vi "Get Available Sets Extended.vi"(8 "error in (no error)":errorcluster, 10 "Item Types (all visible)":T1 items=["all visible", "all including hidden", "standard only", "startup only"], 11 "Session in":refnum<k21>) -> (0 "error out":errorcluster, 2 "Software Sets":T2[](array[typedef]) {"Items"."Visibility Type" items=["standard", "hidden", "system", "unknown", "startup", "image", "essential"]; "Add-ons"."Visibility Type" items=["standard", "hidden", "system", "unknown", "startup", "image", "essential"]}, 3 "Session out":refnum<k21>)   [LabVIEW 2017, in "nisyscfg.lvlib"]
uses:
  <vilib>/nisyscfg/nisyscfg.lvlib
  <vilib>/nisyscfg/Software Set Extended.ctl
  <vilib>/nisyscfg/Software Extended.ctl
  <vilib>/nisyscfg/Component Type.ctl
  <vilib>/nisyscfg/Component Types.ctl
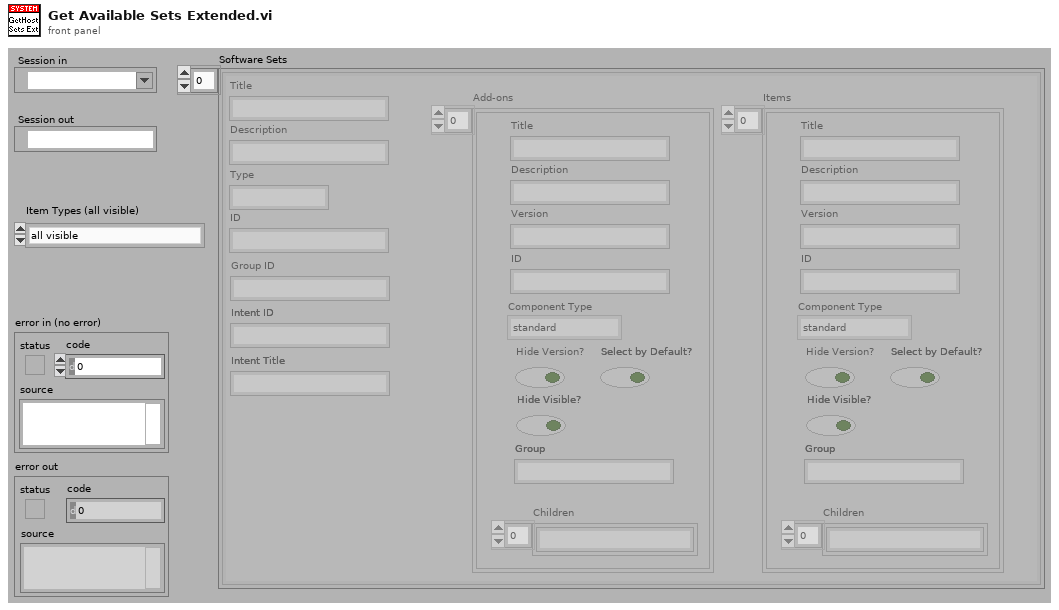
[diagram p1: front panel]
types:
  T1 = typedef "nisyscfg.lvlib/Component Types.ctl" = u32
  T2 = typedef "nisyscfg.lvlib/Software Set Extended.ctl" = cluster{"Description":string, "ID":string, "Type":string, "Title":string, "Add-ons":T3[], "Items":T3[], "Group ID":string, "Intent ID":string, "Intent Title":string}
  T3 = typedef "nisyscfg.lvlib/Software Extended.ctl" = cluster{"Description":string, "ID":string, "Version":string, "Title":string, "Visibility Type":T4, "Hide Version?":bool, "Children":string[], "Select by Default?":bool, "Hide Visible?":bool, "Group":string}
  T4 = typedef "nisyscfg.lvlib/Component Type.ctl" = u32
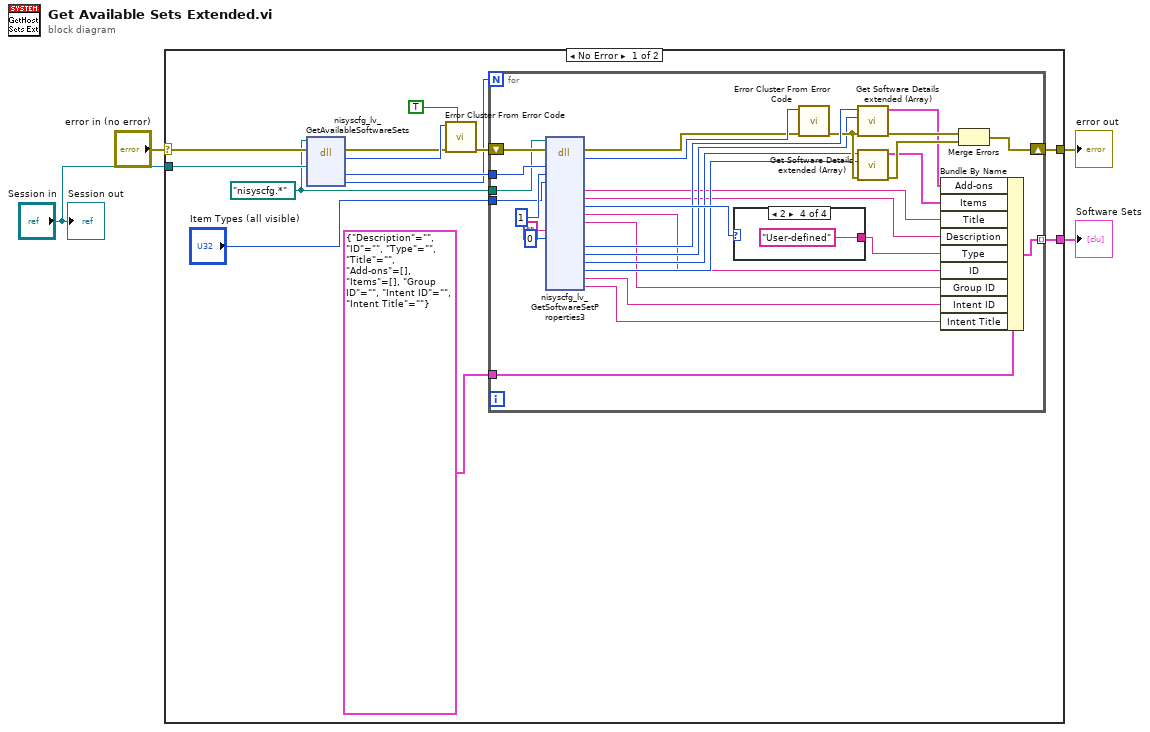
[diagram p0: block diagram]
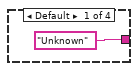
[diagram p2: hidden frame]
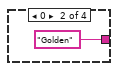
[diagram p3: hidden frame]
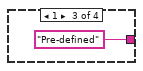
[diagram p4: hidden frame]
diagram:
  n1 = case shown="No Error" "error in (no error)" {
    selector: "error in (no error)" -> [w11 w51]
    tunnel: [w13 w51] -> w4
    tunnel: "Session in" -> [w10 _]
    tunnel: [w12 _] -> w1
    frame No Error {
      w9 = path "nisyscfg.*" ("path in")
      n2 = dll-call lib="nisyscfg.*" fn="nisyscfg_lv_GetAvailableSoftwareSets" label="GetAvailableSoftwareSets"(path in=w9, error in=w11, "system"=w10) -> (error out=w15:errorcluster, "result"=w16:i32, "softwareSets"=w17:u64, "numSets"=w6:i32)  [unwired: 4 in, 1 out]
      n3 = call <vilib>:"Error Cluster From Error Code.vi"("show call chain? (False)"=TRUE, "error in (no error)"=w15, "error code (0)"=w16) -> ("error out"=w14:errorcluster)  [unwired: 6 in]
      n4 = for {
        N: w6 -> [_]
        tunnel: w17 -> [w46]
        shift-right: [w40] -> w13
        shift-left: w14 -> [w45]
        tunnel: T2 {"Description"="", "ID"="", "Type"="", "Title"="", "Add-ons"=[], "Items"=[], "Group ID"="", "Intent ID"="", "Intent Title"=""} ("Software Set") -> [w39]
        tunnel: [w38] -> w12 mode=indexing
        tunnel: w9 -> [w37]
        tunnel: "Item Types (all visible)" -> [w20]
        n5 = dll-call lib="nisyscfg.*" fn="nisyscfg_lv_GetSoftwareSetProperties3" label="GetSoftwareSetProperties3"(path in=w37, error in=w45, "setEnum"=w46, "includeAddOnDeps"=u32 1, "includeTypes"=w20, "version"="", "visibleType"=0) -> (error out=w41:errorcluster, "result"=w42:i32, "title"=w27:string, "description"=w26:string, "type"=w43:u32, "ID"=w24:string, "groupID"=w23:string, "addons"=w36:u64, "numAddons"=w31:i32, "items"=w32:u64, "numItems"=w30:i32, "intentID"=w22:string, "intentTitle"=w21:string)  [unwired: 17 in, 1 out]
        n6 = case shown="2" w43 {
          tunnel: ["Unknown" "Golden" "Pre-defined" "User-defined"] -> w25
          frame Default {
          }
          frame 0 {
          }
          frame 1 {
          }
          frame 2 {
          }
        }
        n7 = call <vilib>:"Error Cluster From Error Code.vi"("error in (no error)"=w41, "error code (0)"=w42) -> ("error out"=w34:errorcluster)  [unwired: 7 in]
        n8 = call <vilib>:"Get Software Details extended (Array).vi"("error in (no error)"=w34, "Number of Elements"=w31, "Enumerator in"=w36) -> ("error out"=w35:errorcluster, "Software Components"=w29:T3[])  [unwired: 7 in]
        n9 = call <vilib>:"Get Software Details extended (Array).vi"("error in (no error)"=w34, "Number of Elements"=w30, "Enumerator in"=w32) -> ("error out"=w33:errorcluster, "Software Components"=w28:T3[])  [unwired: 7 in]
        n10 = Bundle By Name(cluster=w39, "Add-ons"=w29, "Items"=w28, "Title"=w27, "Description"=w26, "Type"=w25, "ID"=w24, "Group ID"=w23, "Intent ID"=w22, "Intent Title"=w21) -> (w38:T2)
        n11 = Merge Errors(w35, w33) -> (w40:errorcluster)
      }
    }
    frame Error {
    }
  }
  "error out" <- w4
  "Software Sets" <- w1
  "Session out" <- "Session in"
